vi "Data To Table.vi"(11 "Data":u8[](array[numeric]) format="%.0x") -> (3 "Array":string[][](array[string]))   [LabVIEW 2021, in "Hex Viewer.lvclass"]
uses:
  Hex Viewer.lvclass
panel:
  out "Processing Time [s]":dbl format="%.3p"
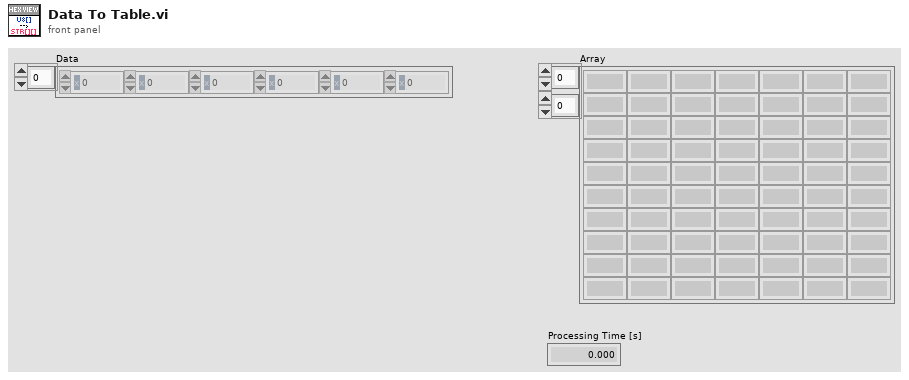
[diagram p1: front panel]
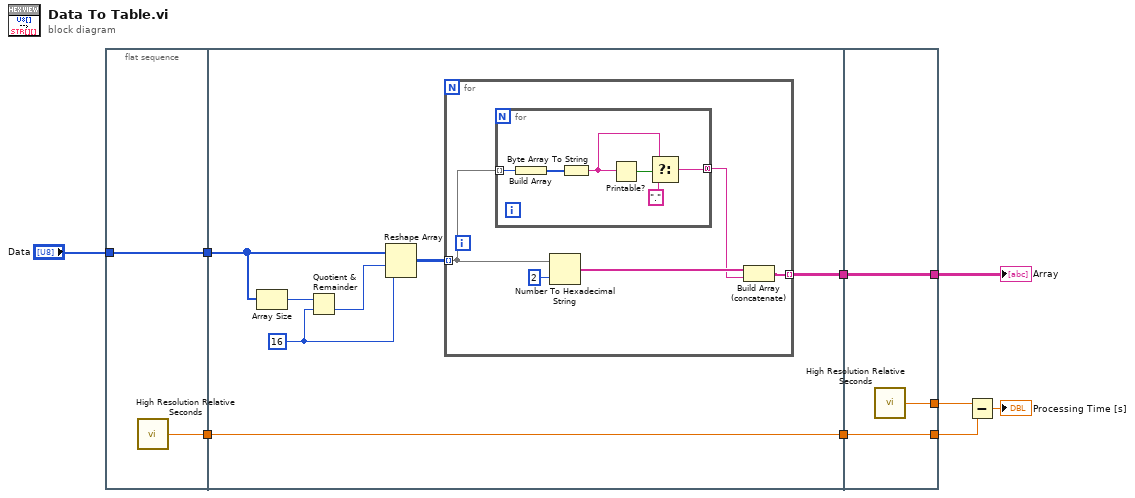
[diagram p0: block diagram]
diagram:
  n1 = flat-sequence {
    tunnel: "Data" -> [w11]
    tunnel: [w11] -> w7
    tunnel: [w10] -> w2
    tunnel: w7 -> [w18]
    tunnel: [w17] -> w6
    tunnel: [w12] -> w3
    tunnel: w2 -> [w12]
    tunnel: [w32] -> w8
    tunnel: w6 -> [w32]
    tunnel: [w31] -> w5
    tunnel: [w30] -> w4
    tunnel: w3 -> [w30]
    frame #0 {
      n2 = call <vilib>:"High Resolution Relative Seconds.vi"() -> ("relative seconds"=w10:dbl)
    }
    frame #1 {
      w15 = 16
      n3 = Array Size(array=w18) -> (size(s)=w14:i32)
      n4 = Quotient & Remainder(x=w14, y=w15) -> (floor(x/y)=w16:i32)  [unwired: 1 out]
      n5 = Reshape Array(w18, w16, w15) -> (w13:u8[][])
      n6 = for {
        tunnel: w13 -> [w20] mode=indexing
        tunnel: [w21] -> w17 mode=indexing
        n7 = for {
          tunnel: w20 -> [w29] mode=indexing
          tunnel: [w24] -> w19 mode=concatenating
          n8 = Build Array(w29) -> (w28:u8[])
          n9 = Byte Array To String(unsigned byte array=w28) -> (string=w26:string)
          n10 = Printable?(1:w26) -> (0:w27:bool)
          n11 = Select(t=w26, s=w27, f=".") -> (s? t:f=w24:string)
        }
        n12 = Number To Hexadecimal String(1:i16 2 ("width (-)"), 2:w20) -> (0:w22:string[])
        n13 = Build Array (concatenate)(w22, w19) -> (w21:string[])
      }
    }
    frame #2 {
      n14 = call <vilib>:"High Resolution Relative Seconds.vi"() -> ("relative seconds"=w31:dbl)
    }
  }
  n15 = Subtract(x=w5, y=w4) -> (x-y=→"Processing Time [s]":dbl)
  "Array" <- w8
